vi "Handle Tab Settings.vi"(6 "Tab Setting Name in":string, 7 "Write? (F:Read)":bool, 8 "error in (no error)":errorcluster, 9 "Tab":refnum<vi>, 11 "Save Restore Settings in":refnum<class "Save Restore Settings.lvclass">) -> (0 "error out":errorcluster, 1 "Sub Controls":T1[](array[typedef]), 3 "Save Restore Settings out":refnum<class "Save Restore Settings.lvclass">)   [LabVIEW 2020, in "Save Restore Settings.lvclass"]
uses:
  <userlib>/_MGI/Application Control/MGI Save Restore Settings/Save Restore Settings.lvclass
  <userlib>/_MGI/Application Control/MGI Save Restore Settings/Control Info.ctl
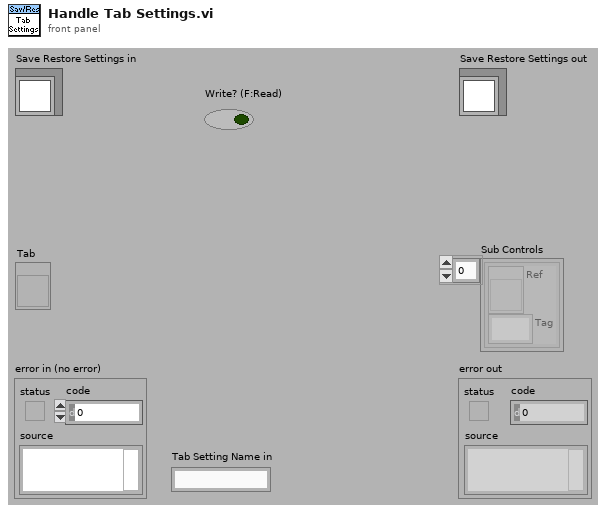
[diagram p1: front panel]
types:
  T1 = typedef "Save Restore Settings.lvclass/Control Info.ctl" = cluster{"Ref":refnum<vi>, "Tag":string}
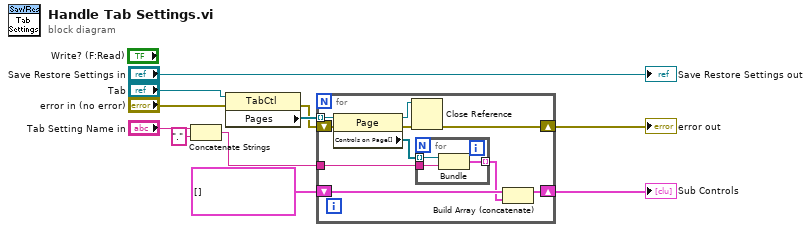
[diagram p0: block diagram]
diagram:
  n1 = Concatenate Strings("Tab Setting Name in", ".") -> (w7:string)
  n2 = property class="TabCtl"(reference="Tab", error in="error in (no error)") -> (error out=w9:errorcluster, "Pages"=w10:refnum<vi>[])  [unwired: 1 out]
  n3 = for {
    tunnel: w10 -> [w21] mode=indexing
    shift-right: [w17] -> w2
    shift-left: w9 -> [w20]
    shift-right: [w13] -> w1
    shift-left: T1[] [] ("Empty 2") -> [w15]
    tunnel: w7 -> [w12]
    n4 = property class="Page"(reference=w21, error in=w20) -> (reference out=w18:refnum<vi>, error out=w19:errorcluster, "Controls on Page[]"=w16:refnum<vi>[])
    n5 = Close Reference(reference=w18, error in (no error)=w19) -> (error out=w17:errorcluster)
    n6 = for {
      tunnel: w16 -> [w22] mode=indexing
      tunnel: [w24] -> w14 mode=indexing
      tunnel: w12 -> [w23]
      n7 = Bundle(w22, w23) -> (w24:cluster{refnum<vi>, string})  [unwired: 1 in]
    }
    n8 = Build Array (concatenate)(w15, w14) -> (w13:T1[])
  }
  "error out" <- w2
  "Sub Controls" <- w1
  "Save Restore Settings out" <- "Save Restore Settings in"
